vi "Done.vi"(8 "error in (no error)":errorcluster, 11 "LVQueue Sink in":refnum<class "LVQueue Sink.lvclass">) -> (0 "error out":errorcluster)   [LabVIEW 2020, in "MVA Framework.lvlib" / "LVQueue Sink.lvclass"]
doc: "--\nCopyright © 2017 Composed SystemsI All rights reserved.\n\nAuthor: Jon McBee <jon.mcbee@composed.io>\n\nThis library is provided \"AS IS\" ,WITHOUT WARRANTIES OR\nCONDITIONS OF ANY KIND, either express or implied.\n\nComposed Systems -- composed.io\n\nStream 0.0.1.1\nJon McBee - Composed Systems\nCopyright (c) 2017, Composed Systems"
uses:
  LVQueue Sink.lvclass
  LVQueue Sink.lvclass/LVQueue Sink.ctl
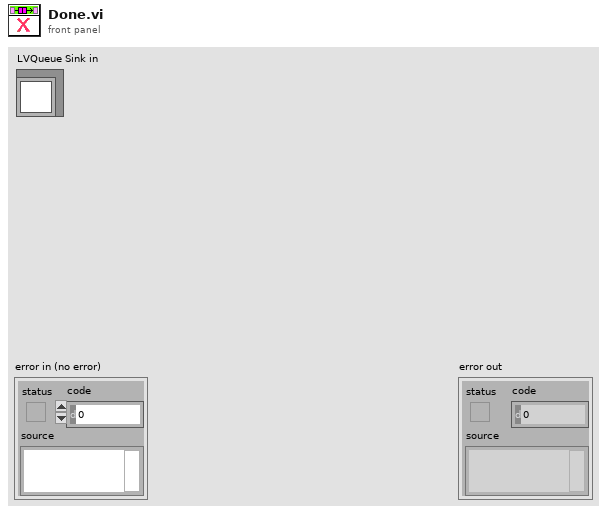
[diagram p1: front panel]
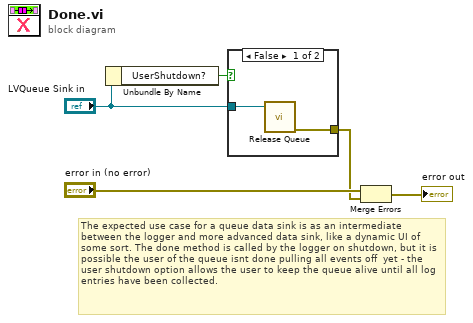
[diagram p0: block diagram]
diagram:
  # "The expected use case for a queue data sink is as an intermediate between the logger and more advanced data sink, like a dynamic UI of some sort. The done method is called by the logger on shutdown, but it is possible the user of the queue isnt done pulling all events off  yet - the user shutdown option allows the user to keep the queue alive until all log entries have been collected."
  n1 = Unbundle By Name("LVQueue Sink in") -> ("UserShutdown?"=w3:bool)
  n2 = case shown="False" w3 {
    tunnel: "LVQueue Sink in" -> [w7 _]
    tunnel: [w6 _] -> w1
    frame False {
      n3 = call "Release Queue.vi"("LVQueue Sink in"=w7) -> ("error out"=w6:errorcluster)  [unwired: 9 in, 1 out]
    }
    frame True {
    }
  }
  n4 = Merge Errors("error in (no error)", w1) -> (→"error out":errorcluster)
